vi "TCP控制代码.vi"(0 "发送内容：":string, 1 "timeout ms (wait forever: -1)":i32=-1 caption="超时毫秒（一直等待:-1）", 5 "发送按钮":bool, 7 "端口号 2":u16=6342 caption="端口", 9 "停止运行":bool caption="停止", 11 "ledoff":bool, 12 "ledon":bool) -> (4 "remote address":string caption="控制器ip", 6 "接收数据":string)   [LabVIEW 2016]
panel:
  out "错误输出":errorcluster
  out "接收:":string caption="接收数据："
  in  "清除接收":bool
  in  "清除发送":bool
  in  "端口号":u16=6342 caption="端口"
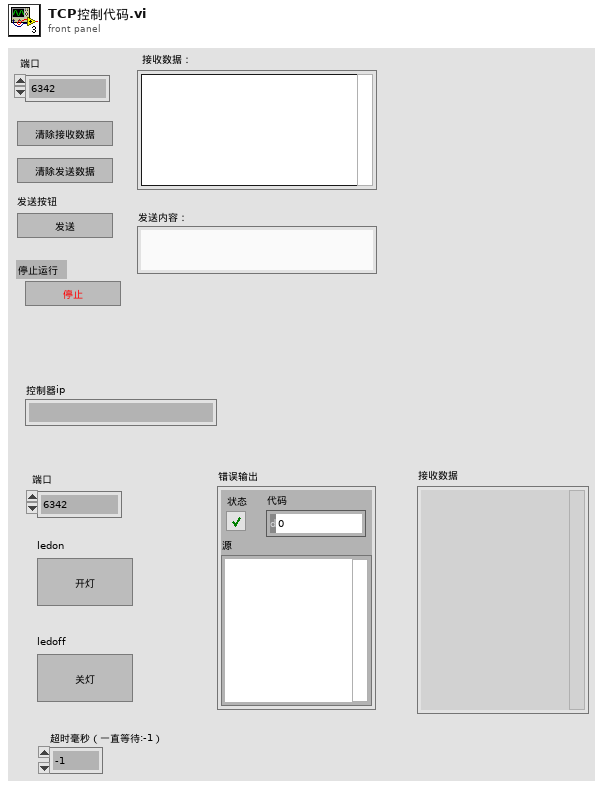
[diagram p1: front panel]
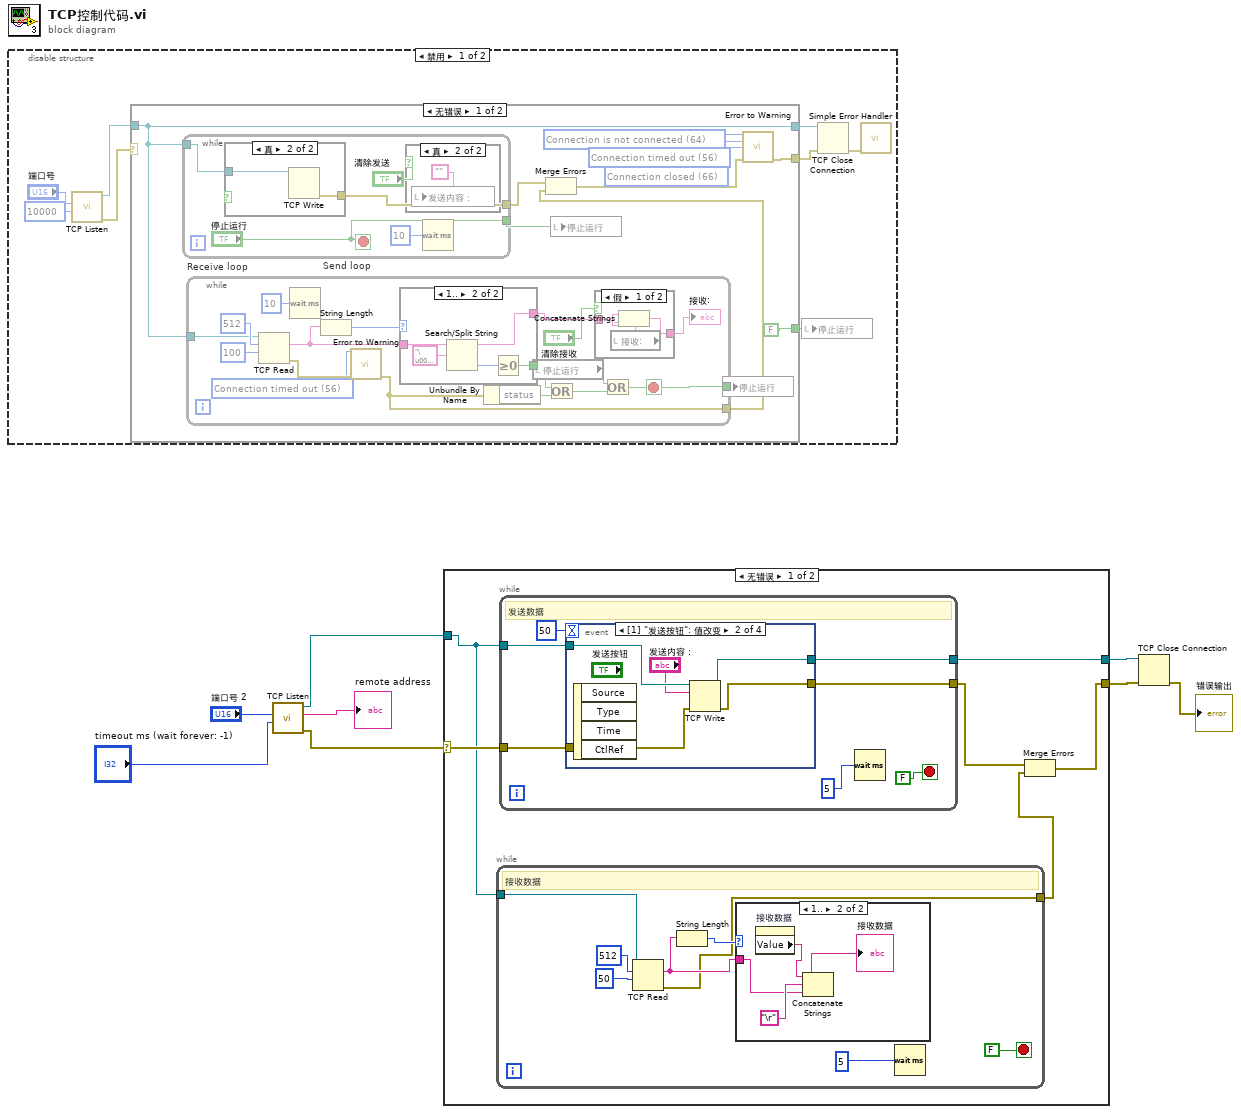
[diagram p0: block diagram]
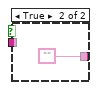
[diagram p4: hidden frame]
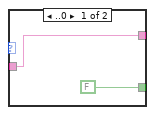
[diagram p5: hidden frame]
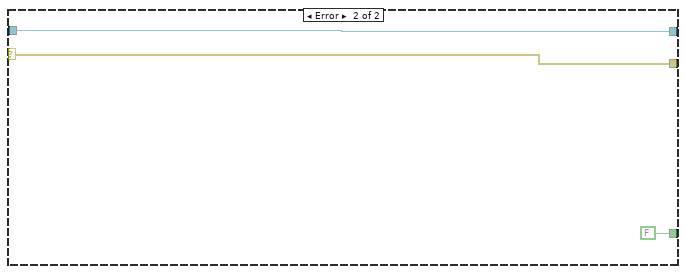
[diagram p6: hidden frame]
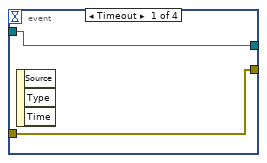
[diagram p9: hidden frame]
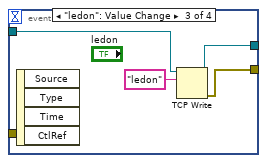
[diagram p10: hidden frame]
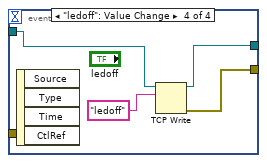
[diagram p11: hidden frame]
diagram:
  n1 = disable-structure shown="禁用" {
    frame Disabled {
      n2 = call <vilib>:"TCP Listen.vi"("timeout ms (wait forever: -1)"=10000, "port"="端口号") -> ("error out"=w9:errorcluster, "connection ID"=w10:refnum<k5>)  [unwired: 5 in, 3 out]
      n3 = case shown="无错误" w9 {
        selector: w9 -> [_ w66]
        tunnel: [w21 w66] -> w12
        tunnel: w10 -> [w27 w67]
        tunnel: [w27 w67] -> w11
        tunnel: [FALSE FALSE] -> w14
        frame No Error {
          w18 = 56 items=["No Error", "Argument Error", "Memory Full", "Out of Zone", "End of File", "File Already Open", "Generic File IO Error", "File Not Found", "File Permission Error", "Disk Full", "Duplicate Path", "Too Many Files Open", "Not Enabled", "Resource File Not Found", "Cannot Add Resource", "Resource Not Found", "Image Not Found", "Image Memory Error", "Pen Does Not Exist", "Config Bad Type", "Config Token Not Found", "Config Parse Error", "Config Memory Error", "Bad External Code Format", "Bad External Code Offset", "External Code Not Present", "Null Window", "Destroy Window Mixup", "Null Menu", "Print Aborted", "Bad Print Record", "Print Driver Error", "Windows Error During Print", "Memory Error During Print", "Print Dialog Error", "Generic Print Error", "Invalid Device Refnum", "Device Not Found", "Device Parameter Error", "Device Unit Error", "Can't Open Device", "Device Call Aborted", "Generic Error", "Cancelled By User", "Object ID Too Low", "Object ID Too High", "Object Not In Heap", "Unknown Heap", "Bad DefProc ID", "DefProc Not In Table", "Message Out Of Range", "Null Method", "Unknown Message", "Manager Call Not Supported", "Bad address", "Connection In progress", "Connection timed out", "Connection is already in progress", "Network attribute not supported", "Network error", "Address in use", "System out of memory", "Connection aborted", "Connection refused", "Connection is not connected", "Connection is already connected", "Connection closed", "Initialize error (interapplication manager)", "Bad occurrence", "Wait on unbound occurrence handler", "Occurrence queue overflow", "Bad path", "Semaphore not signaled", "Unrecognized type (interapplication manager)"] ("2nd Error to Convert")
          w22 = 66 items=["No Error", "Argument Error", "Memory Full", "Out of Zone", "End of File", "File Already Open", "Generic File IO Error", "File Not Found", "File Permission Error", "Disk Full", "Duplicate Path", "Too Many Files Open", "Not Enabled", "Resource File Not Found", "Cannot Add Resource", "Resource Not Found", "Image Not Found", "Image Memory Error", "Pen Does Not Exist", "Config Bad Type", "Config Token Not Found", "Config Parse Error", "Config Memory Error", "Bad External Code Format", "Bad External Code Offset", "External Code Not Present", "Null Window", "Destroy Window Mixup", "Null Menu", "Print Aborted", "Bad Print Record", "Print Driver Error", "Windows Error During Print", "Memory Error During Print", "Print Dialog Error", "Generic Print Error", "Invalid Device Refnum", "Device Not Found", "Device Parameter Error", "Device Unit Error", "Can't Open Device", "Device Call Aborted", "Generic Error", "Cancelled By User", "Object ID Too Low", "Object ID Too High", "Object Not In Heap", "Unknown Heap", "Bad DefProc ID", "DefProc Not In Table", "Message Out Of Range", "Null Method", "Unknown Message", "Manager Call Not Supported", "Bad address", "Connection In progress", "Connection timed out", "Connection is already in progress", "Network attribute not supported", "Network error", "Address in use", "System out of memory", "Connection aborted", "Connection refused", "Connection is not connected", "Connection is already connected", "Connection closed", "Initialize error (interapplication manager)", "Bad occurrence", "Wait on unbound occurrence handler", "Occurrence queue overflow", "Bad path", "Semaphore not signaled", "Unrecognized type (interapplication manager)"] ("3rd Error to Convert")
          w23 = 64 items=["No Error", "Argument Error", "Memory Full", "Out of Zone", "End of File", "File Already Open", "Generic File IO Error", "File Not Found", "File Permission Error", "Disk Full", "Duplicate Path", "Too Many Files Open", "Not Enabled", "Resource File Not Found", "Cannot Add Resource", "Resource Not Found", "Image Not Found", "Image Memory Error", "Pen Does Not Exist", "Config Bad Type", "Config Token Not Found", "Config Parse Error", "Config Memory Error", "Bad External Code Format", "Bad External Code Offset", "External Code Not Present", "Null Window", "Destroy Window Mixup", "Null Menu", "Print Aborted", "Bad Print Record", "Print Driver Error", "Windows Error During Print", "Memory Error During Print", "Print Dialog Error", "Generic Print Error", "Invalid Device Refnum", "Device Not Found", "Device Parameter Error", "Device Unit Error", "Can't Open Device", "Device Call Aborted", "Generic Error", "Cancelled By User", "Object ID Too Low", "Object ID Too High", "Object Not In Heap", "Unknown Heap", "Bad DefProc ID", "DefProc Not In Table", "Message Out Of Range", "Null Method", "Unknown Message", "Manager Call Not Supported", "Bad address", "Connection In progress", "Connection timed out", "Connection is already in progress", "Network attribute not supported", "Network error", "Address in use", "System out of memory", "Connection aborted", "Connection refused", "Connection is not connected", "Connection is already connected", "Connection closed", "Initialize error (interapplication manager)", "Bad occurrence", "Wait on unbound occurrence handler", "Occurrence queue overflow", "Bad path", "Semaphore not signaled", "Unrecognized type (interapplication manager)"] ("1st Error to Convert")
          n4 = while "Send loop" {
            tunnel: w27 -> [w33]
            tunnel: ["停止运行"] -> w19
            tunnel: [w32] -> w25
            stop <- "停止运行" stop-if-true
            n5 = case shown="真" w31 {
              tunnel: [_ w36] -> w32
              tunnel: w33 -> [_ w35]
              frame False {
              }
              frame True {
                n6 = TCP Write(connection ID=w35) -> (error out=w36:errorcluster)  [unwired: 3 in, 2 out]
              }
            }
            n7 = case shown="真" "清除发送" {
              frame False {
              }
              frame True {
                n8 = local write "发送内容："("") -> ()
              }
            }
            n9 = Wait (ms)(milliseconds to wait=u32 10 ("等待时间（毫秒）")) -> ()  [unwired: 1 out]
          }
          n10 = while "Receive loop" {
            tunnel: [w50] -> w20
            tunnel: [w44] -> w26
            tunnel: w27 -> [w51]
            stop <- w50 stop-if-true
            w45 = 56 items=["No Error", "Argument Error", "Memory Full", "Out of Zone", "End of File", "File Already Open", "Generic File IO Error", "File Not Found", "File Permission Error", "Disk Full", "Duplicate Path", "Too Many Files Open", "Not Enabled", "Resource File Not Found", "Cannot Add Resource", "Resource Not Found", "Image Not Found", "Image Memory Error", "Pen Does Not Exist", "Config Bad Type", "Config Token Not Found", "Config Parse Error", "Config Memory Error", "Bad External Code Format", "Bad External Code Offset", "External Code Not Present", "Null Window", "Destroy Window Mixup", "Null Menu", "Print Aborted", "Bad Print Record", "Print Driver Error", "Windows Error During Print", "Memory Error During Print", "Print Dialog Error", "Generic Print Error", "Invalid Device Refnum", "Device Not Found", "Device Parameter Error", "Device Unit Error", "Can't Open Device", "Device Call Aborted", "Generic Error", "Cancelled By User", "Object ID Too Low", "Object ID Too High", "Object Not In Heap", "Unknown Heap", "Bad DefProc ID", "DefProc Not In Table", "Message Out Of Range", "Null Method", "Unknown Message", "Manager Call Not Supported", "Bad address", "Connection In progress", "Connection timed out", "Connection is already in progress", "Network attribute not supported", "Network error", "Address in use", "System out of memory", "Connection aborted", "Connection refused", "Connection is not connected", "Connection is already connected", "Connection closed", "Initialize error (interapplication manager)", "Bad occurrence", "Wait on unbound occurrence handler", "Occurrence queue overflow", "Bad path", "Semaphore not signaled", "Unrecognized type (interapplication manager)"] ("1st Error to Convert")
            n11 = TCP Read(connection ID=w51, bytes to read=512, 9:100) -> (data out=w49:string, error out=w46:errorcluster)  [unwired: 2 in, 1 out]
            n12 = Wait (ms)(milliseconds to wait=u32 10 ("等待时间（毫秒）")) -> ()  [unwired: 1 out]
            n13 = String Length(string=w49) -> (length=w53:i32)
            n14 = call <vilib>:"Error to Warning.vi"("1st Error to Convert"=w45, "error in"=w46) -> ("warning out"=w44:errorcluster)  [unwired: 13 in]
            n15 = case shown="1.." w53 {
              tunnel: w49 -> [w58 w63]
              tunnel: [w58 w60] -> w38
              tunnel: [FALSE w61] -> w48
              frame ..0 {
              }
              frame 1.. {
                n16 = Search/Split String(string=w63, search string/char (-)="\u0004") -> (substring before match=w60:string, offset of match=w62:i32)  [unwired: 1 in, 1 out]
                n17 = Greater Or Equal To 0?(x=w62) -> (x >= 0?=w61:bool)
              }
            }
            n18 = Unbundle By Name(w44) -> ("status"=w43:bool)
            n19 = local read "停止运行"() -> (w42:bool)
            n20 = Or(x=w48, y=w43) -> (x .or. y?=w41:bool)
            n21 = case shown="假" "清除接收" {
              tunnel: [w54 ""] -> w39
              tunnel: w38 -> [w55 _]
              frame False {
                n22 = local read "接收:"() -> (w56:string)
                n23 = Concatenate Strings(w56, w55) -> (w54:string)
              }
              frame True {
              }
            }
            "接收:" <- w39
            n24 = Or(x=w42, y=w41) -> (x .or. y?=w50:bool)
          }
          n25 = Merge Errors(w25, w26) -> (w24:errorcluster)
          n26 = local write "停止运行"(w19) -> ()
          n27 = local write "停止运行"(w20) -> ()
          n28 = call <vilib>:"Error to Warning.vi"("1st Error to Convert"=w23, "2nd Error to Convert"=w18, "3rd Error to Convert"=w22, "error in"=w24) -> ("warning out"=w21:errorcluster)  [unwired: 11 in]
        }
        frame Error {
        }
      }
      n29 = local write "停止运行"(w14) -> ()
      n30 = TCP Close Connection(connection ID=w11, error in (no error)=w12) -> (error out=w13:errorcluster)  [unwired: 1 in, 1 out]
      n31 = call <vilib>:"Simple Error Handler.vi"("error in (no error)"=w13) -> ()  [unwired: 4 in, 5 out]
    }
    frame Enabled {
    }
  }
  n32 = call <vilib>:"TCP Listen.vi"("timeout ms (wait forever: -1)"="timeout ms (wait forever: -1)", "port"="端口号 2") -> ("error out"=w6:errorcluster, "remote address"=→"remote address":string, "connection ID"=w5:refnum<k5>)  [unwired: 5 in, 2 out]
  n33 = case shown="无错误" w6 {
    selector: w6 -> [w72 w108]
    tunnel: w5 -> [w71 w109]
    tunnel: [w69 w108] -> w3
    tunnel: [w73 w109] -> w2
    frame No Error {
      n34 = while {
        tunnel: w71 -> [w77]
        tunnel: [w74] -> w68
        stop <- FALSE stop-if-true
        # "接收数据"
        n35 = TCP Read(connection ID=w77, bytes to read=512, 9:50) -> (data out=w75:string, error out=w74:errorcluster)  [unwired: 2 in, 1 out]
        n36 = String Length(string=w75) -> (length=w76:i32)
        n37 = case shown="1.." w76 {
          tunnel: w75 -> [_ w82]
          frame ..0 {
          }
          frame 1.. {
            n38 = property on="接收数据" class="Str"() -> ("Value"=w84:string)  [unwired: 2 in, 2 out]
            n39 = Concatenate Strings(w84, "\r", w82) -> (→"接收数据":string)
          }
        }
        n40 = Wait (ms)(milliseconds to wait=u32 5 ("等待时间（毫秒）")) -> ()  [unwired: 1 out]
      }
      n41 = while {
        tunnel: w71 -> [w90]
        tunnel: [w89] -> w70
        tunnel: [w88] -> w73
        tunnel: w72 -> [w87]
        stop <- FALSE stop-if-true
        # "发送数据"
        n42 = event shown="[1] \"发送按钮\": 值改变" {
          selector: _ -> [_ _ _ _]
          dyn-events: _ -> [_ _ _ _]
          timeout: 50 -> [_ _ _ _]
          tunnel: w90 -> [w94 w97 w103 w106]
          tunnel: [w93 w99 w101 w104] -> w89
          tunnel: [w94 w98 w100 w105] -> w88
          tunnel: w87 -> [w93 w96 _ _]
          event Timeout {
            n43 = event-data() -> ()  [unwired: 1 in, 3 out]
          }
          event "发送按钮": Value Change {
            n44 = event-data() -> ()  [unwired: 1 in, 4 out]
            n45 = TCP Write(connection ID=w97, data in="发送内容：", error in (no error)=w96) -> (connection ID out=w98:refnum<k5>, error out=w99:errorcluster)  [unwired: 1 in, 1 out]
          }
          event "ledon": Value Change {
            n46 = event-data() -> ()  [unwired: 1 in, 4 out]
            n47 = TCP Write(connection ID=w103, data in="ledon" ("数据输入")) -> (connection ID out=w100:refnum<k5>, error out=w101:errorcluster)  [unwired: 2 in, 1 out]
          }
          event "ledoff": Value Change {
            n48 = event-data() -> ()  [unwired: 1 in, 4 out]
            n49 = TCP Write(connection ID=w106, data in="ledoff" ("数据输入")) -> (connection ID out=w105:refnum<k5>, error out=w104:errorcluster)  [unwired: 2 in, 1 out]
          }
        }
        n50 = Wait (ms)(milliseconds to wait=u32 5 ("等待时间（毫秒）")) -> ()  [unwired: 1 out]
      }
      n51 = Merge Errors(w70, w68) -> (w69:errorcluster)
    }
    frame Error {
    }
  }
  n52 = TCP Close Connection(connection ID=w2, error in (no error)=w3) -> (error out=→"错误输出":errorcluster)  [unwired: 1 in, 1 out]
